vi "RT_init_vars.vi"(0 "connection parameters":T1={"baud rate (9600)"=115200, "data bits (8)"=8, "stop bits (10: 1 bit)"=10, "parity (0:none)"=enum."None", "flow control (0:none)"=0, "timeout (10sec)"=10000, "Enable Termination\nChar (T)"=TRUE, "termination char\n(0xA = '\\n' = LF)\n(0xD = '\\r' = CF) "=13} {"stop bits (10: 1 bit)" items=["1.0"=10, "1.5"=15, "2.0"=20]; "flow control (0:none)" items=["None", "XON/XOFF", "RTS/CTS", "XON/XOFF & RTS/CTS", "DTR/DSR", "XON/XOFF & DTR/DSR"]}) -> (2 "FPGA VI Reference Out":refnum<k20>, 3 "FPGA I/O IRQ Number(s)":i32, 4 "port name out":refnum<visa-resource-name>, 5 "error out":errorcluster)   [LabVIEW 2018]
uses:
  Globals/RT Stop.vi
  Globals/RT AND FPGA SETTINGS.vi
  <vilib>/FPGAPlugInAG/cRIO-9074/niLvFpga_Open_cRIO-9074.vi
  <vilib>/rvi/interface/common/dynamic/niFpgaDynamicAddResources.vi
  <vilib>/FPGAPlugInAG/Dynamic/niLvFpga_Reset_Dynamic.vi
  <vilib>/FPGAPlugInAG/Dynamic/niLvFpga_Run_Dynamic.vi
  <vilib>/Utility/error.llb/Error Cluster From Error Code.vi
  <vilib>/rvi/errors/niLvFpgaAdjustHostInterfaceError.vi
  <vilib>/rvi/interface/nirviOpenFPGA/nirviOpenFPGA.xnode
  FPGA Bitfiles/remotecontroller_FPGATarget_FPGAMain_RhGo+c1SRDI.lvbitx
  FPGA Main.vi
  <vilib>/rvi/interface/nirviMethod/nirviMethod.xnode
  <vilib>/rvi/interface/nirviReadWriteControl/nirviReadWriteControl.xnode
  <vilib>/rvi/interface/Simulation/niFpgaSimulationCallBeginRW.vi
  NiFpgaLv.dll
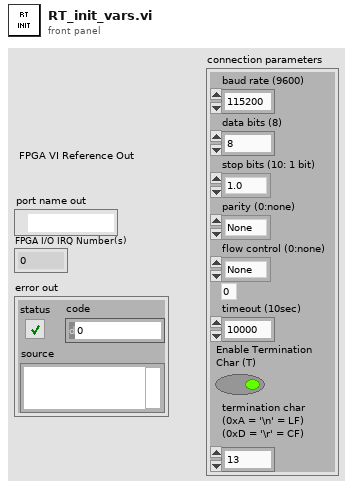
[diagram p1: front panel]
types:
  T1 = cluster{"baud rate (9600)":u32, "data bits (8)":u16, "stop bits (10: 1 bit)":u16, "parity (0:none)":enum16{"None", "Odd", "Even", "Mark", "Space"}, "flow control (0:none)":u16, "timeout (10sec)":u32, "Enable Termination\nChar (T)":bool, "termination char\n(0xA = '\\n' = LF)\n(0xD = '\\r' = CF) ":u8}
  T2 = cluster{"2: expecting response?":bool, "expected max length":u32}
  T3 = cluster{"1: do writing?":bool, "write buffer":string}
  T4 = cluster{"0. connect/reconnect?":bool, "last: disconnect?":bool, "slow serial port init delay":u32}
  T5 = enum16{"Safe State", "I/O with PID Control", "Fast Output Only", "NOT_READY"}
  T6 = enum8{"High Speed", "Best 60 Hz Rejection", "Best 50 Hz Rejection", "High Resolution"}
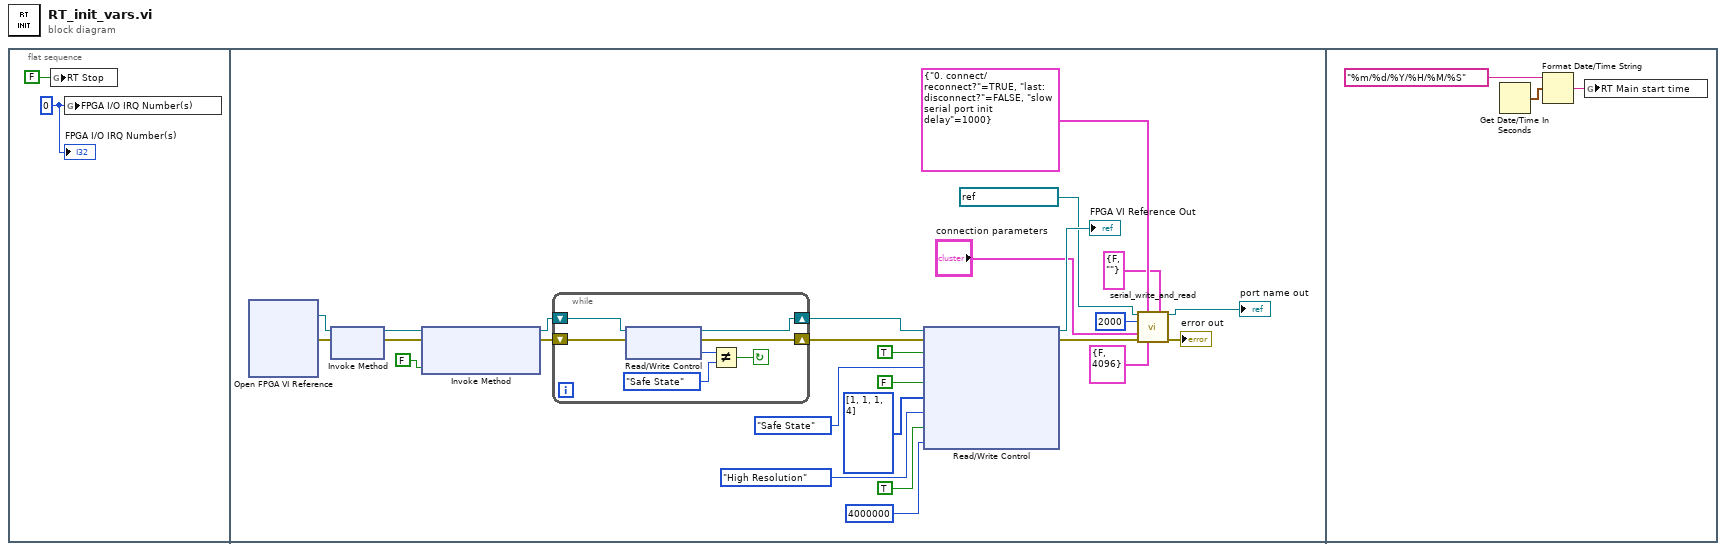
[diagram p0: block diagram]
diagram:
  n1 = flat-sequence {
    frame #0 {
      w2 = 0 ("FPGA I/O IRQ Number(s)")
      n2 = global write "RT Stop.vi" "RT Stop"(FALSE ("RT Stop")) -> ()
      n3 = global write "RT AND FPGA SETTINGS.vi" "FPGA I/O IRQ Number(s)"(w2) -> ()
      "FPGA I/O IRQ Number(s)" <- w2
    }
    frame #1 {
      n4 = xnode "Open FPGA VI Reference"() -> ("FPGA VI Reference Out"=w22:refnum<k20>, "error out"=w23:errorcluster)  [unwired: 2 in]
      n5 = xnode "Invoke Method"("FPGA VI Reference In"=w22, "error in"=w23) -> ("FPGA VI Reference Out"=w15:refnum<k20>, "error out"=w14:errorcluster)
      n6 = xnode "Invoke Method"("FPGA VI Reference In"=w15, "error in"=w14, "Wait Until Done (F)"=FALSE) -> ("FPGA VI Reference Out"=w13:refnum<k20>, "error out"=w11:errorcluster)
      n7 = while {
        shift-right: [w34] -> w12
        shift-left: w13 -> [w35]
        shift-right: [w32] -> w10
        shift-left: w11 -> [w33]
        stop <- w29 continue-if-true
        n8 = xnode "Read/Write Control"("FPGA VI Reference In"=w35, "error in"=w33) -> ("FPGA VI Reference Out"=w34:refnum<k20>, "error out"=w32:errorcluster, "FPGA state"=w31:T5)
        n9 = Not Equal?(x=w31, y=T5."Safe State") -> (x != y?=w29:bool)
      }
      n10 = xnode "Read/Write Control"("FPGA VI Reference In"=w12, "error in"=w10, "RTMain Running?"=TRUE, "FPGA state"=T5."Safe State", "Enable Watchdog"=FALSE, "Input voltage range"=u8[] [1, 1, 1, 4], "9219 Conversion Time"=T6."High Resolution", "Update  9219 settings"=TRUE ("Update 9219 settings"), "ticks"=i64 4000000) -> ("FPGA VI Reference Out"=→"FPGA VI Reference Out":refnum<k20>, "error out"=w18:errorcluster)
      n11 = call "serial_write_and_read.vi"("port name in"=refnum<visa-resource-name> "ASRL1::INSTR", "0 and last: Connection/Reconnection setting"=T4 {"0. connect/reconnect?"=TRUE, "last: disconnect?"=FALSE, "slow serial port init delay"=1000}, "1. writing setting input"=T3 {"1: do writing?"=FALSE, "write buffer"=""}, "total operation timeout (ms)"=u32 2000 ("timeout (ms)"), "connection parameters"="connection parameters", "error in"=w18, "2. reading settings input"=T2 {"2: expecting response?"=FALSE, "expected max length"=4096}) -> ("port name out"=→"port name out":refnum<visa-resource-name>, "error out"=→"error out":errorcluster)  [unwired: 6 in, 1 out]
    }
    frame #2 {
      n12 = Get Date/Time In Seconds() -> (seconds since 1Jan1904=w38:timestamp)
      n13 = Format Date/Time String(time format string (%c)="%m/%d/%Y/%H/%M/%S", seconds (now)=w38) -> (date/time string=w36:string)  [unwired: 1 in]
      n14 = global write "RT AND FPGA SETTINGS.vi" "RT Main start time"(w36) -> ()
    }
  }
